vi "Terminla_GearSystem_Work_Condition.vi"() -> ()   [LabVIEW 2014]
panel:
  out "达到工作条件":bool
  in  "齿轮子系统监测参数":T1
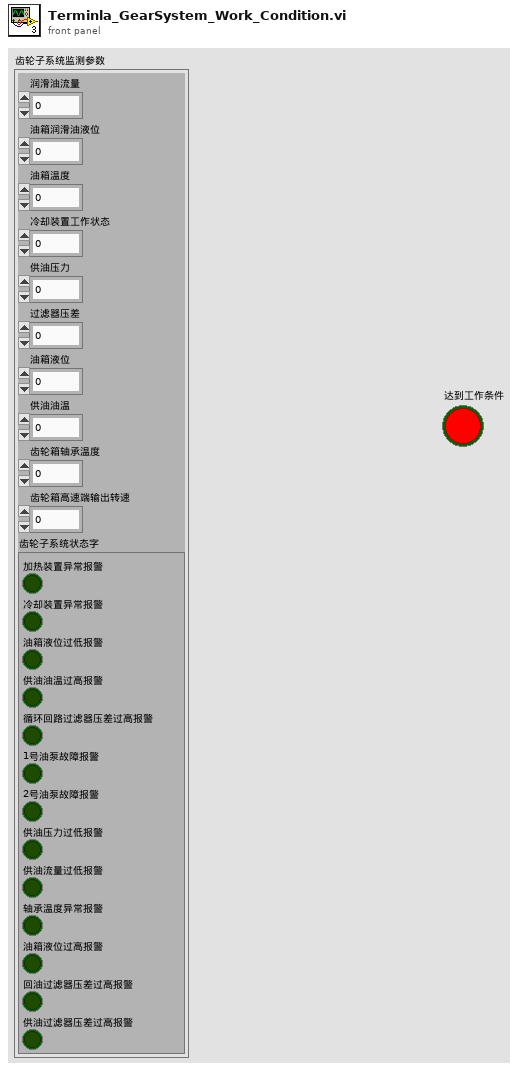
[diagram p1: front panel]
types:
  T1 = cluster{"润滑油流量":u16, "油箱润滑油液位":u16, "油箱温度":u16, "冷却装置工作状态":u16, "供油压力":u16, "过滤器压差":u16, "油箱液位":u16, "供油油温":u16, "齿轮箱轴承温度":u16, "齿轮箱高速端输出转速":u16, "齿轮子系统状态字":cluster{"加热装置异常报警":bool, "冷却装置异常报警":bool, "油箱液位过低报警":bool, "供油油温过高报警":bool, "循环回路过滤器压差过高报警":bool, "1号油泵故障报警":bool, "2号油泵故障报警":bool, "供油压力过低报警":bool, "供油流量过低报警":bool, "轴承温度异常报警":bool, "油箱液位过高报警":bool, "回油过滤器压差过高报警":bool, "供油过滤器压差过高报警":bool}}
  T2 = cluster{"加热装置异常报警":bool, "冷却装置异常报警":bool, "油箱液位过低报警":bool, "供油油温过高报警":bool, "循环回路过滤器压差过高报警":bool, "1号油泵故障报警":bool, "2号油泵故障报警":bool, "供油压力过低报警":bool, "供油流量过低报警":bool, "轴承温度异常报警":bool, "油箱液位过高报警":bool, "回油过滤器压差过高报警":bool, "供油过滤器压差过高报警":bool}
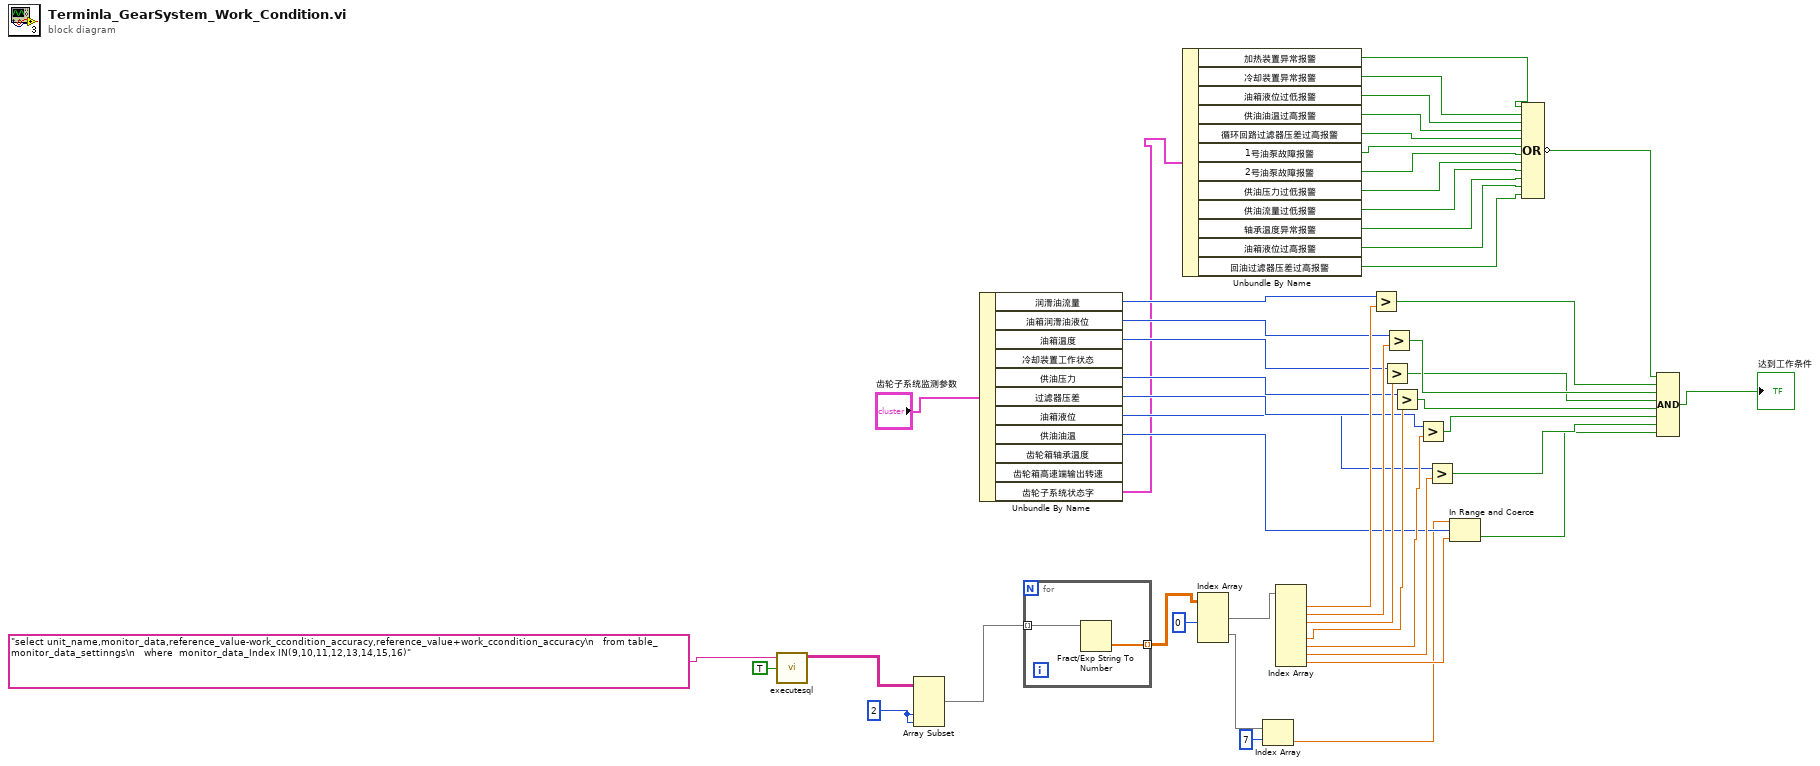
[diagram p0: block diagram]
diagram:
  w46 = 2
  n1 = call "executesql.vi"("Return Data (T)"=TRUE, "Command Text"="select unit_name,monitor_data,reference_value-work_ccondition_accuracy,reference_value+work_ccondition_accuracy\n   from table_monitor_data_settinngs\n   where  monitor_data_Index IN(9,10,11,12,13,14,15,16)") -> ("Data"=w33:string[][])  [unwired: 5 in, 1 out]
  n2 = Array Subset(array=w33, index (col)=w46, length (col)=w46) -> (w45:string[][])  [unwired: 2 in]
  n3 = Unbundle By Name("齿轮子系统监测参数") -> ("润滑油流量"=w40:u16, "油箱润滑油液位"=w38:u16, "油箱温度"=w36:u16, "供油压力"=w34:u16, "过滤器压差"=w31:u16, "油箱液位"=w29:u16, "供油油温"=w27:u16, "齿轮子系统状态字"=w15:T2)  [unwired: 3 out]
  n4 = for {
    tunnel: w45 -> [w50] mode=indexing
    tunnel: [w49] -> w44 mode=indexing
    n5 = Fract/Exp String To Number(string=w50) -> (number=w49:dbl[])  [unwired: 3 in, 1 out]
  }
  n6 = Unbundle By Name(w15) -> ("加热装置异常报警"=w14:bool, "冷却装置异常报警"=w13:bool, "油箱液位过低报警"=w12:bool, "供油油温过高报警"=w11:bool, "循环回路过滤器压差过高报警"=w10:bool, "1号油泵故障报警"=w9:bool, "2号油泵故障报警"=w8:bool, "供油压力过低报警"=w7:bool, "供油流量过低报警"=w6:bool, "轴承温度异常报警"=w5:bool, "油箱液位过高报警"=w4:bool, "回油过滤器压差过高报警"=w3:bool)
  n7 = Index Array(array=w44, index (col) #1=0) -> (element #1=w42:dbl[], element #2=w41:dbl[])  [unwired: 3 in]
  n8 = Index Array(array=w41, index=7) -> (element=w24:dbl)
  n9 = Index Array(array=w42) -> (element #1=w39:dbl, element #2=w37:dbl, element #3=w35:dbl, element #5=w32:dbl, element #6=w30:dbl, element #7=w28:dbl, element #8=w26:dbl)  [unwired: 8 in, 1 out]
  n10 = Greater?(x=w40, y=w39) -> (0:w23:bool)
  n11 = Greater?(x=w36, y=w35) -> (0:w21:bool)
  n12 = Greater?(x=w38, y=w37) -> (0:w22:bool)
  n13 = Greater?(x=w34, y=w32) -> (0:w20:bool)
  n14 = Greater?(x=w31, y=w30) -> (0:w19:bool)
  n15 = Greater?(x=w29, y=w28) -> (0:w18:bool)
  n16 = In Range and Coerce(upper limit=w24, x=w27, lower limit=w26) -> (In Range?=w17:bool)  [unwired: 1 out]
  n17 = Compound Arithmetic op=OR(w14, w13, w12, w11, w10, w9, w8, w7, w6, w5, w4, w3) -> (invert w2:bool)
  n18 = Compound Arithmetic op=AND(w2, w23, w22, w21, w20, w19, w18, w17) -> (→"达到工作条件":bool)
